vi "Decimate Array.vi"(8 "error in (no error)":errorcluster, 10 "decimating factor (1)":i32=1, 11 "XY-data":cluster{"X-array":dbl[], "Y-array":dbl[]}[](array[cluster]) {"Y-array" format="%.2p"; "X-array" format="%.2p"}) -> (0 "error out":errorcluster, 3 "Decimated XY-data out":cluster{"X-array":dbl[], "Y-array":dbl[]}[](array[cluster]) {"Y-array" format="%.2p"; "X-array" format="%.2p"})   [LabVIEW 2019, in "xy_utilities.lvlib"]
doc: "Decimates the input <b>XY-data</b> by the <b>decimating factor</b>."
uses:
  xy_utilities.lvlib
  <vilib>/Analysis/NI_AALPro.lvlib
  <vilib>/Analysis/2dsp.llb/Decimate (single shot, DBL).vi
  _OpenG.lib/array/array.llb/Delete Elements from 1D Array (Variant)__ogtk.vi
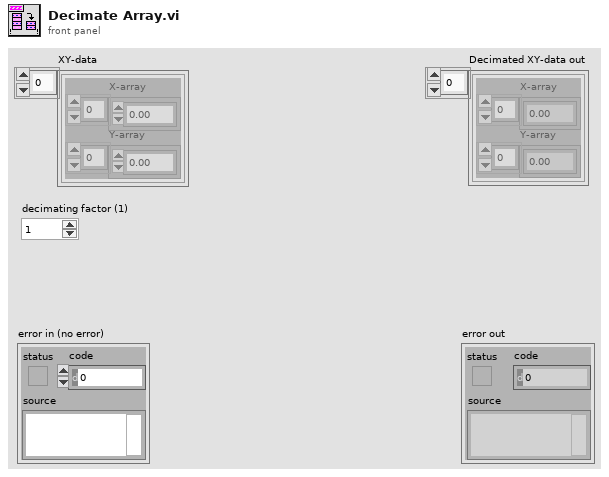
[diagram p1: front panel]
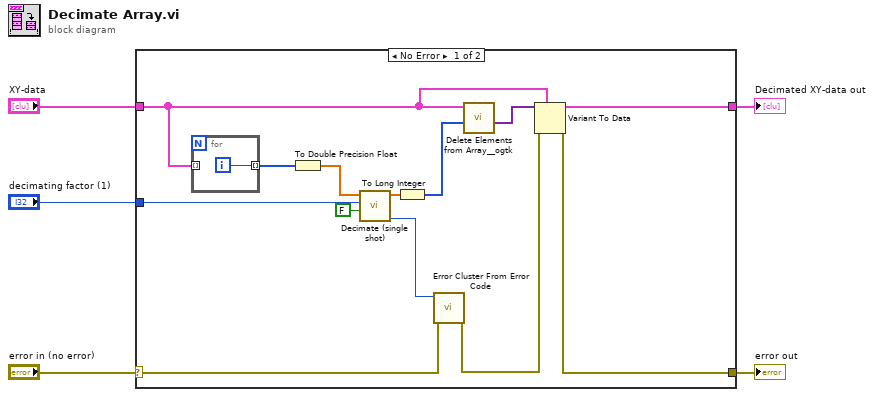
[diagram p0: block diagram]
diagram:
  n1 = case shown="No Error" "error in (no error)" {
    selector: "error in (no error)" -> [w14 w21]
    tunnel: "XY-data" -> [w6 w20]
    tunnel: [w7 w20] -> w3
    tunnel: [w8 w21] -> w2
    tunnel: "decimating factor (1)" -> [w18 _]
    frame No Error {
      n2 = for {
        tunnel: w6 -> [_] mode=indexing
        tunnel: [w19] -> w16 mode=indexing
        i -> [w19]
      }
      n3 = To Double Precision Float(number=w16) -> (double precision float=w11:dbl[])
      n4 = call-poly <vilib>:"Decimate (single shot).vi"("averaging"=FALSE, "decimating factor"=w18, "X"=w11) -> ("error"=w15:i32, "Decimated Array"=w13:dbl[])  [unwired: 7 in]
      n5 = To Long Integer(number=w13) -> (32bit integer=w12:i32[])
      n6 = call <vilib>:"Error Cluster From Error Code.vi"("error in (no error)"=w14, "error code (0)"=w15) -> ("error out"=w9:errorcluster)  [unwired: 7 in]
      n7 = call-poly "Delete Elements from Array__ogtk.vi"("indices"=w12, "array"=w6) -> ("deleted elements"=w10:variant[])  [unwired: 8 in, 1 out]
      n8 = Variant To Data(error in=w9, type=w6, Variant=w10) -> (data=w7:cluster{"X-array":dbl[], "Y-array":dbl[]}[], error out=w8:errorcluster)
    }
    frame Error {
    }
  }
  "error out" <- w2
  "Decimated XY-data out" <- w3
